vi "FPGA Globals.vi"() -> ()   [LabVIEW 2020]
uses:
  TypeDef/FPGA Settings.ctl
  TypeDef/FPGA_DAQ_settings.ctl
  TypeDef/FPGA_adapter_type.ctl
  TypeDef/FPGA_card_type.ctl
panel:
  out "FPGA DAQ Settings":T1
  out "System MAC Addresses":string[](array[string])
  in  "FPGA System Settings":T4={"System Clock(MHz)"=240.0, "FPGA MAC 1"="AABBCCDDEEFF", "Port Number 1"=1, "Port Number 2"=2, "FPGA MAC 2"="AABBCCDDEEFF", "PC MAC Address"=""}
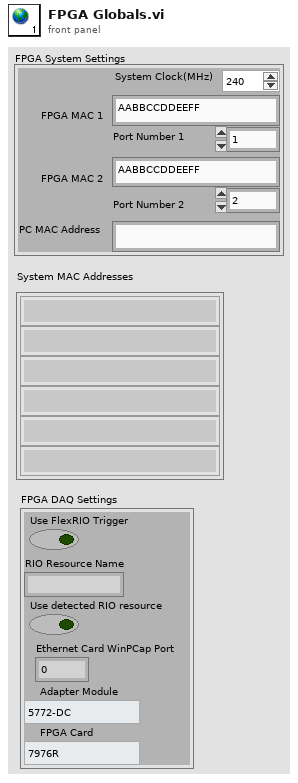
[diagram p1: front panel]
types:
  T1 = typedef "FPGA_DAQ_settings.ctl" = cluster{"Use FlexRIO Trigger":bool, "RIO Resource Name":string, "Use detected RIO resource":bool, "Ethernet Card WinPCap Port ":i16, "Adapter Module":T2, "FPGA Card":T3}
  T2 = typedef "FPGA_adapter_type.ctl" = enum16{"5772-DC", "5772-AC"}
  T3 = typedef "FPGA_card_type.ctl" = enum16{"7976R", "7975R", "7966R"}
  T4 = typedef "FPGA Settings.ctl" = cluster{"System Clock(MHz)":dbl, "FPGA MAC 1":string, "Port Number 1":i32, "Port Number 2":i32, "FPGA MAC 2":string, "PC MAC Address":string}
diagram:
